vi "Install Script.vi"(8 "error in (no error)":errorcluster) -> (0 "error out":errorcluster)   [LabVIEW 2014]
uses:
  <vilib>/Utility/miscctls.llb/LVPointTypeDef.ctl
panel:
  out "path":path
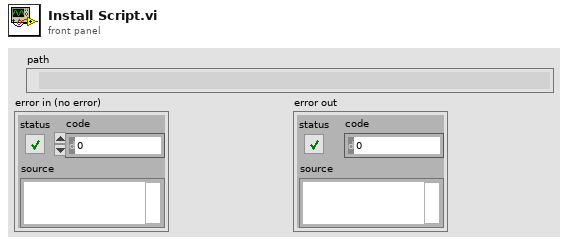
[diagram p1: front panel]
types:
  T1 = typedef "LVPointTypeDef.ctl" = cluster{"Horizontal":i16, "Vertical":i16}
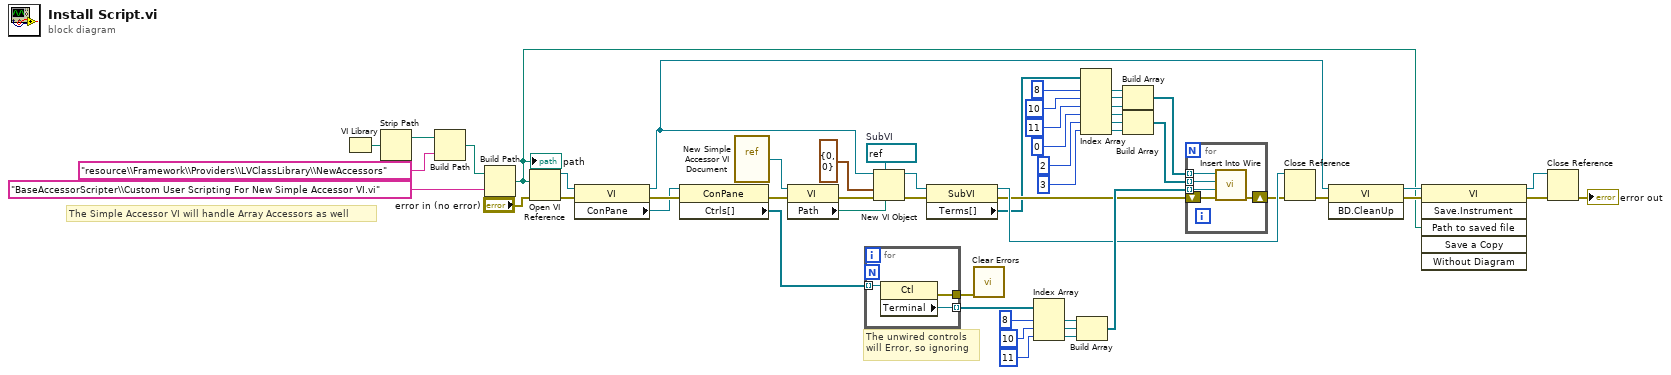
[diagram p0: block diagram]
diagram:
  w23 = refnum<vi> refnum  # SubVI
  # "The Simple Accessor VI will handle Array Accessors as well"
  # "The unwired controls\nwill Error, so ignoring"
  n1 = VI Library() -> (path=w54:path)
  n2 = Strip Path(path=w54) -> (stripped path=w53:path)  [unwired: 1 out]
  n3 = Build Path(base path=w53, name or relative path="resource\\Framework\\Providers\\LVClassLibrary\\NewAccessors") -> (appended path=w51:path)
  n4 = Build Path(base path=w51, name or relative path="BaseAccessorScripter\\Custom User Scripting For New Simple Accessor VI.vi") -> (appended path=w3:path)
  "path" <- w3
  n5 = Open VI Reference(vi path=w3, error in (no error)="error in (no error)") -> (vi reference=w14:refnum<vi>, error out=w47:errorcluster)  [unwired: 4 in]
  n6 = property class="VI"(reference=w14, error in=w47) -> (reference out=w8:refnum<vi>, error out=w20:errorcluster, "ConPane"=w15:refnum<vi>)
  n7 = property class="ConPane"(reference=w15, error in=w20) -> (error out=w48:errorcluster, "Ctrls[]"=w18:refnum<vi>[])  [unwired: 1 out]
  n8 = vi-ref "New Simple Accessor VI Document.vi"() -> (w13:refnum<vi>)
  n9 = property class="VI"(reference=w13, error in=w48) -> (error out=w49:errorcluster, "Path"=w21:path)  [unwired: 1 out]
  n10 = for {
    tunnel: w18 -> [w57] mode=indexing
    tunnel: [w56] -> w19 mode=indexing
    tunnel: [w55] -> w46
    n11 = property class="Ctl"(reference=w57) -> (error out=w55:errorcluster, "Terminal"=w56:refnum<vi>)  [unwired: 1 in, 1 out]
  }
  n12 = New VI Object(vi object class=w23, owner refnum=w8, position/next to=T1 {"Horizontal"=0, "Vertical"=0} ("location"), 6:w21, 8:w49) -> (object refnum=w22:refnum<vi>, 0:w32:errorcluster)  [unwired: 3 in]
  n13 = property class="SubVI"(reference=w22, error in=w32) -> (reference out=w35:refnum<vi>, error out=w33:errorcluster, "Terms[]"=w24:refnum<vi>[])
  n14 = call <vilib>:"Clear Errors.vi"("error in (no error)"=w46) -> ()  [unwired: 5 in, 2 out]
  n15 = Index Array(array=w19, index #1=8 ("index"), index #2=10 ("index"), index #3=11 ("index")) -> (element #1=w36:refnum<vi>, element #2=w37:refnum<vi>, element #3=w38:refnum<vi>)
  n16 = Build Array(w36, w37, w38) -> (w45:refnum<vi>[])
  n17 = Index Array(array=w24, index #1=8 ("index"), index #2=10 ("index"), index #3=11 ("index"), index #4=0 ("index"), index #5=2 ("index"), index #6=3 ("index")) -> (element #1=w42:refnum<vi>, element #2=w43:refnum<vi>, element #3=w44:refnum<vi>, element #4=w39:refnum<vi>, element #5=w40:refnum<vi>, element #6=w41:refnum<vi>)
  n18 = Build Array(w42, w43, w44) -> (w9:refnum<vi>[])
  n19 = Build Array(w39, w40, w41) -> (w10:refnum<vi>[])
  n20 = for {
    shift-right: [w62] -> w7
    shift-left: w33 -> [w58]
    tunnel: w45 -> [w59] mode=indexing
    tunnel: w9 -> [w61] mode=indexing
    tunnel: w10 -> [w60] mode=indexing
    n21 = call "Insert Into Wire.vi"("error in (no error)"=w58, "Wire Source Term"=w59, "Output Term"=w60, "Input Term"=w61) -> ("error out"=w62:errorcluster)  [unwired: 7 in]
  }
  n22 = Close Reference(reference=w35, error in (no error)=w7) -> (error out=w6:errorcluster)
  n23 = invoke class="VI" method="BD.CleanUp"(reference=w8, error in=w6) -> (reference out=w5:refnum<vi>, error out=w4:errorcluster)  [unwired: 1 in, 1 out]
  n24 = invoke class="VI" method="Save.Instrument"(reference=w5, error in=w4, "Path to saved file"=w3) -> (reference out=w1:refnum<vi>, error out=w2:errorcluster)  [unwired: 3 in, 4 out]
  n25 = Close Reference(reference=w1, error in (no error)=w2) -> (error out=→"error out":errorcluster)
